vi "SystemLink_Write_Boolean.vi"(9 "Boolean":bool, 11 "SL_XControl":string(xcontrol)) -> ()   [LabVIEW 2020]
uses:
  SL_XControl.xctl
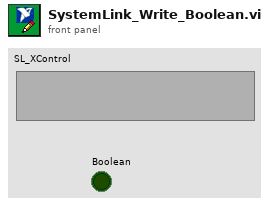
[diagram p1: front panel]
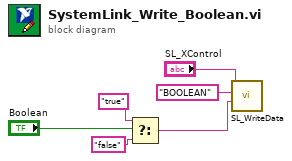
[diagram p0: block diagram]
diagram:
  n1 = Select(t="true", s="Boolean", f="false") -> (s? t:f=w1:string)
  n2 = call "SL_WriteData.vi"("Data"=w1, "Type"="BOOLEAN", "Path"="SL_XControl") -> ()  [unwired: 9 in]
